vi "Change tab page colour.vi"(7 "Action":T1(ring), 8 "error in (no error)":errorcluster, 9 "New Colour":u32(colorbox), 10 "Page Indices":i32[](array[numeric]), 11 "TabControl in":refnum<vi>) -> (0 "error out":errorcluster)   [LabVIEW 2012]
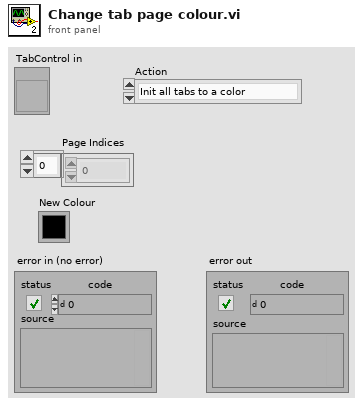
[diagram p1: front panel]
types:
  T1 = enum16{"Init all tabs to a color", "Change specific tabs"}
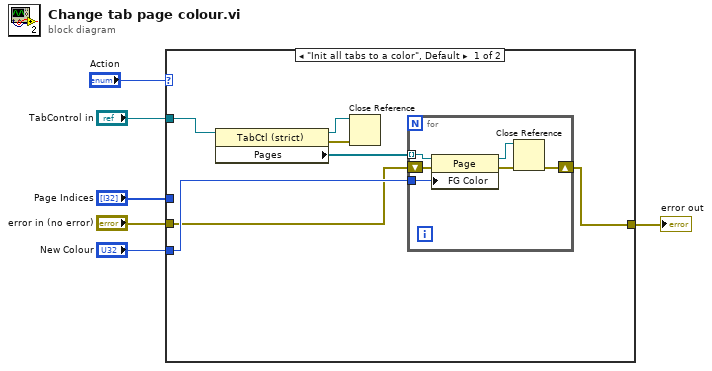
[diagram p0: block diagram]
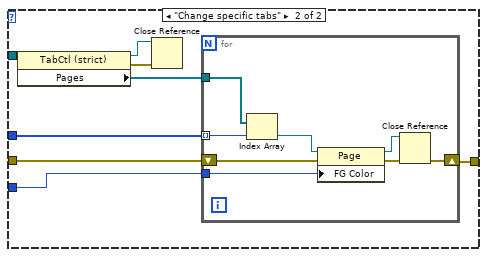
[diagram p2: hidden frame]
diagram:
  n1 = case shown="\"Init all tabs to a color\", Default" "Action" {
    tunnel: "New Colour" -> [w9 w27]
    tunnel: "TabControl in" -> [w11 w24]
    tunnel: "Page Indices" -> [_ w22]
    tunnel: [w7 w21] -> w3
    tunnel: "error in (no error)" -> [w8 w20]
    frame "Init all tabs to a color", Default {
      n2 = property class="TabCtl (strict)"(reference=w11) -> (reference out=w13:refnum<vi>, error out=w12:errorcluster, "Pages"=w10:refnum<vi>[])  [unwired: 1 in]
      n3 = Close Reference(reference=w13, error in (no error)=w12) -> ()  [unwired: 1 out]
      n4 = for {
        tunnel: w10 -> [w17] mode=indexing
        tunnel: w9 -> [w16]
        shift-right: [w14] -> w7
        shift-left: w8 -> [w15]
        n5 = property class="Page"(reference=w17, error in=w15, "FG Color"=w16) -> (reference out=w19:refnum<vi>, error out=w18:errorcluster)
        n6 = Close Reference(reference=w19, error in (no error)=w18) -> (error out=w14:errorcluster)
      }
    }
    frame "Change specific tabs" {
      n7 = property class="TabCtl (strict)"(reference=w24) -> (reference out=w26:refnum<vi>, error out=w25:errorcluster, "Pages"=w23:refnum<vi>[])  [unwired: 1 in]
      n8 = Close Reference(reference=w26, error in (no error)=w25) -> ()  [unwired: 1 out]
      n9 = for {
        tunnel: w27 -> [w33]
        tunnel: w23 -> [w32]
        tunnel: w22 -> [w31] mode=indexing
        shift-right: [w30] -> w21
        shift-left: w20 -> [w29]
        n10 = Index Array(array=w32, index=w31) -> (element=w28:refnum<vi>)
        n11 = property class="Page"(reference=w28, error in=w29, "FG Color"=w33) -> (reference out=w35:refnum<vi>, error out=w34:errorcluster)
        n12 = Close Reference(reference=w35, error in (no error)=w34) -> (error out=w30:errorcluster)
      }
    }
  }
  "error out" <- w3
